vi "2D Convolution (CDB).vi"(8 "output size":enum32{"full", "size X", "compact"}(ring), 9 "algorithm":enum32{"direct", "frequency domain"}(ring)=enum."frequency domain", 10 "Y":cdb[][](array[numeric]), 11 "X":cdb[][](array[numeric])) -> (0 "error":i32, 3 "X * Y":cdb[][](array[numeric]))   [LabVIEW 2020, in "NI_AALPro.lvlib"]
doc: "Computes the convolution of the input sequences <B>X</B> and <B>Y</B>. Wire data to the <B>X</B> and <B>Y</B> inputs to determine the polymorphic instance to use or manually select the instance."
uses:
  <vilib>/Analysis/NI_AALPro.lvlib
  <resource>/lvanlys.dll
panel:
  # "2D Convolution (CDB)"
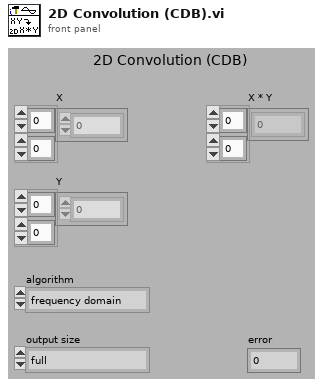
[diagram p1: front panel]
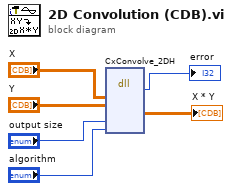
[diagram p0: block diagram]
diagram:
  n1 = dll-call lib="e:/builds/penguin/labview/branches/2020/dev/dist/resource/lvanlys.*" fn="CxConvolve_2DH"("X"="X", "Y"="Y", "size"="output size", "domain"="algorithm") -> (→"error":i32, "X * Y"=→"X * Y":cdb[][])  [unwired: 8 in, 2 out]
